vi "test input FG.vi"(1 "Test Controls":T1 {"Slider" scale=0.0..10.0}, 2 "Menu":T2) -> (0 "Test Controls Out":T1 {"Slider" scale=0.0..10.0})   [LabVIEW 2014]
uses:
  typedefs/fg_getset.ctl
  typedefs/test/test controls.ctl
panel:
  # "Stores Data for Test Inputs"
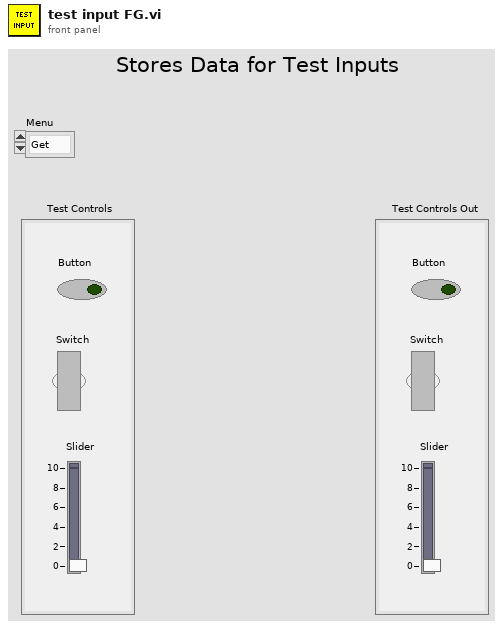
[diagram p1: front panel]
types:
  T1 = typedef "test controls.ctl" = cluster{"Button":bool, "Switch":bool, "Slider":dbl}
  T2 = typedef "fg_getset.ctl" = enum16{"Get", "Set"}
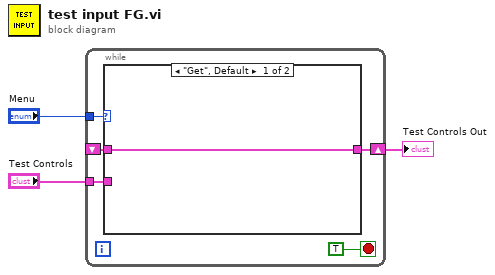
[diagram p0: block diagram]
diagram:
  n1 = while {
    tunnel: "Menu" -> [w8]
    tunnel: "Test Controls" -> [w6]
    shift-right: [w5] -> w1
    shift-left: _ -> [w4]
    stop <- TRUE stop-if-true
    n2 = case shown="\"Get\", Default" w8 {
      tunnel: w6 -> [_ w10]
      tunnel: [w9 w10] -> w5
      tunnel: w4 -> [w9 _]
      frame "Get", Default {
      }
      frame "Set" {
      }
    }
  }
  "Test Controls Out" <- w1
